vi "CalcStdErrFit.vi"(6 "Weight":dbl[](array[numeric]), 7 "Y":dbl[](array[numeric]), 8 "error in":errorcluster, 9 "covariance":T1, 10 "Best Fit Params":dbl[](array[numeric]) format="%#.10g", 11 "best nonlinear fit":dbl[](array[numeric])) -> (0 "error out":errorcluster, 1 "std error":dbl[](array[numeric]) format="%#.10g", 2 "R-square":dbl)   [LabVIEW 2018]
uses:
  <vilib>/Analysis/Matrix/Datatypes/RealMatrix.ctl
  <vilib>/Analysis/NI_AALPro.lvlib
  <vilib>/Analysis/Matrix/NI_Matrix.lvlib
panel:
  out "DOF":i32
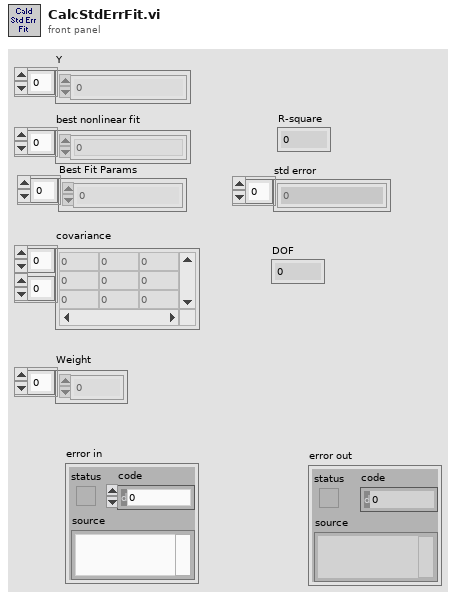
[diagram p1: front panel]
types:
  T1 = typedef "NI_Matrix.lvlib/RealMatrix.ctl" = dbl[][]
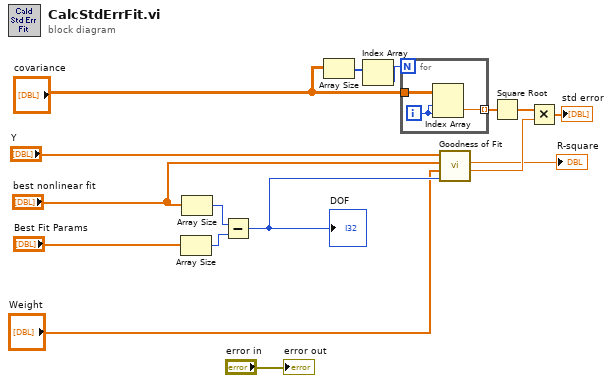
[diagram p0: block diagram]
diagram:
  n1 = Array Size(array="Best Fit Params") -> (size(s)=w7:i32)
  n2 = Array Size(array="best nonlinear fit") -> (size(s)=w6:i32)
  n3 = Subtract(x=w6, y=w7) -> (x-y=w5:i32)
  "DOF" <- w5
  n4 = Array Size(array="covariance") -> (size(s)=w15:i32[])
  n5 = Index Array(array=w15) -> (element=w14:i32)  [unwired: 1 in]
  n6 = for {
    N: w14 -> [_]
    tunnel: "covariance" -> [w19]
    tunnel: [w17] -> w13 mode=indexing
    i -> [w18]
    n7 = Index Array(array=w19, index (row)=w18, index (col)=w18) -> (element=w17:dbl)
  }
  n8 = call <vilib>:"Goodness of Fit.vi"("degree of freedom"=w5, "Weight"="Weight", "Best Fit"="best nonlinear fit", "Y"="Y") -> ("RMSE"=w11:dbl, "R-square"=→"R-square":dbl)  [unwired: 4 in, 2 out]
  n9 = Square Root(x=w13) -> (sqrt(x)=w10:dbl[])
  n10 = Multiply(x=w10, y=w11) -> (x*y=→"std error":dbl[])
  "error out" <- "error in"
